vi "M14_Turret_Hardware_Begin.vi"   [LabVIEW 2019]
uses:
  M14 Turret_Hardware_Globals.vi
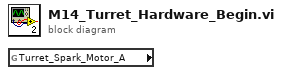
[diagram p0: block diagram]
diagram:
  n1 = global read "M14 Turret_Hardware_Globals.vi" "Turret_Spark_Motor_A"() -> ()  [unwired: 1 out]
